vi "COPD_labview.vi"() -> ()   [LabVIEW 2022 SP3]
uses:
  <vilib>/DAQmx/read.llb/DAQmx Read (Analog DBL 1Chan 1Samp).vi
  <vilib>/Instr/_visa.llb/VISA Configure Serial Port (Instr).vi
  <vilib>/DAQmx/create/channels.llb/DAQmx Create Channel (AI-Voltage-Basic).vi
  <vilib>/DAQmx/miscellaneous.llb/DAQmx Fill In Error Info.vi
panel:
  out "Visa out":string
  out "Centered Piezo Chart":dbl(graph)
  in  "Peizo Baseline":dbl
  out "Command Sent":string
  in  "ESP32 COM Port":refnum<visa-resource-name>
  out "Bed Motor ON":bool
  out "Oxygen Relay ON":bool
  out "SpO2 Danger":bool
  out "Oxygen Required":bool
  in  "Danger Threshold":dbl
  out "SpO2 Chart":dbl(graph)
  out "SpO2  (%)":dbl
  in  "Oxygen Threshold":dbl
  out "Fever Alert":bool
  in  "Temperature Threshold":dbl
  out "Temperature(C) Indicator":dbl
  out "Temperature Chart":dbl(graph)
  in  "Breath Threshold":dbl
  in  "stop":bool
  out "Breath Detected":bool
  out "Piezo Signal Chart":dbl(graph)
  out "Respiratory Rate":dbl
  out "Piezo Voltage":dbl
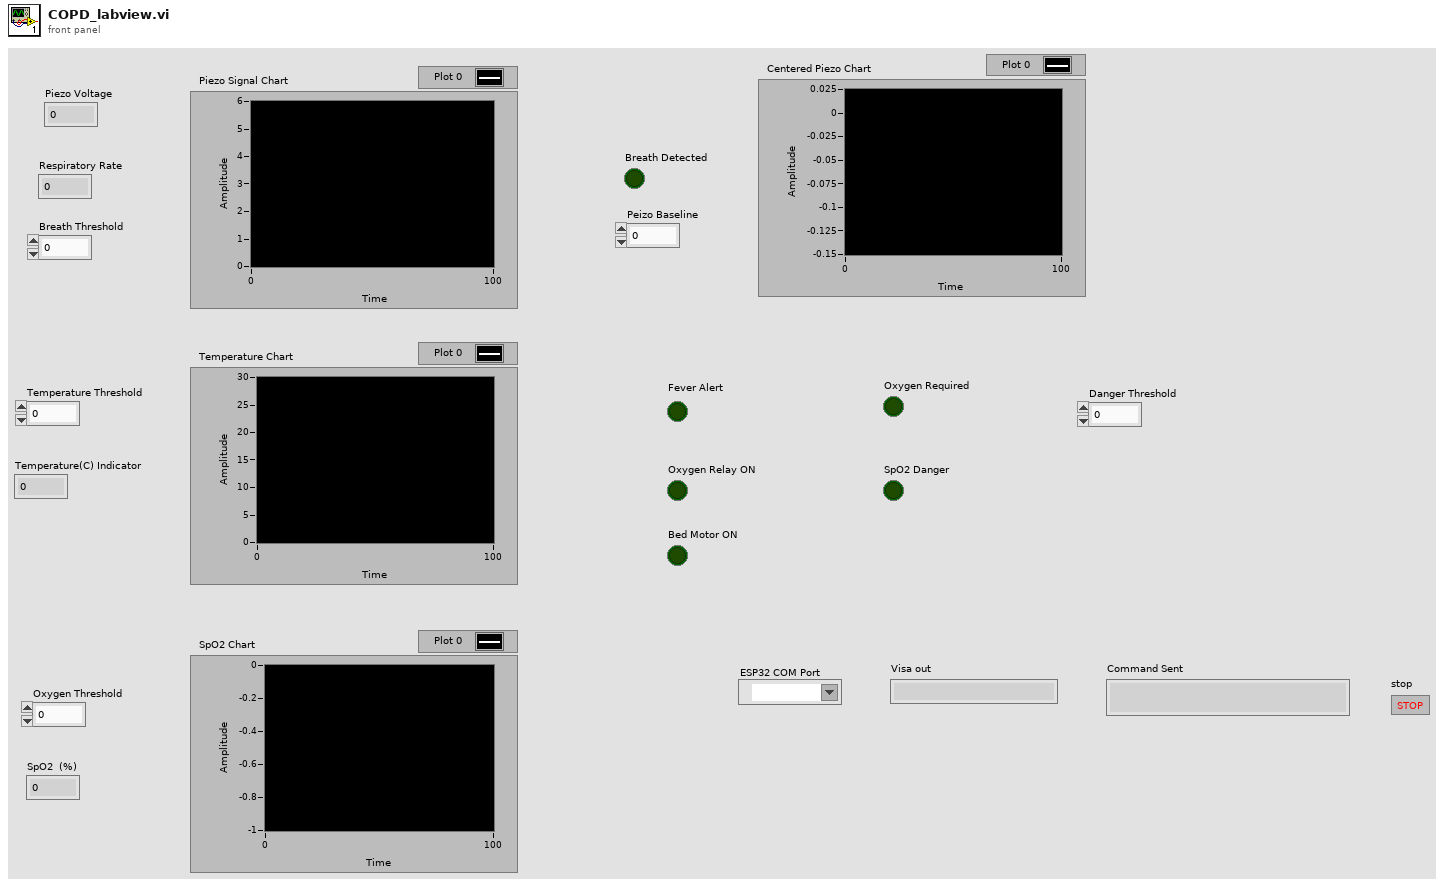
[diagram p1: front panel]
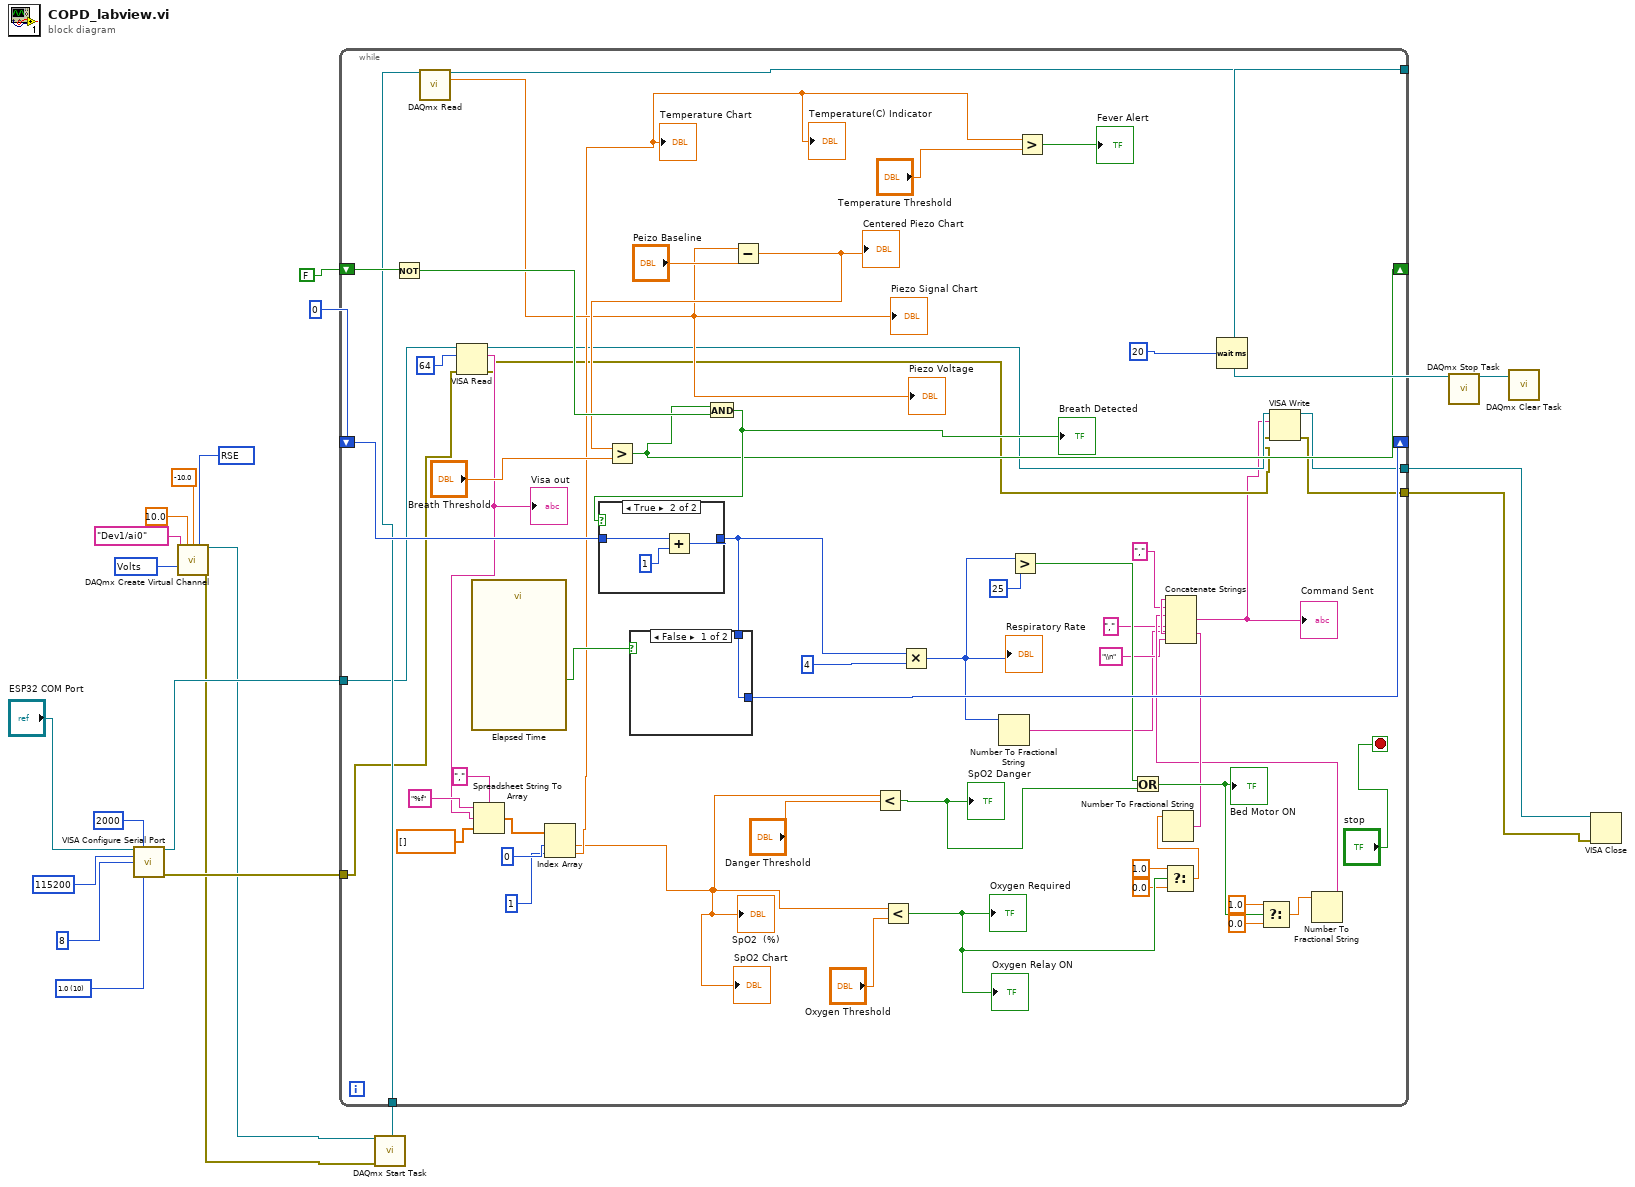
[diagram p0: block diagram]
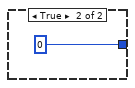
[diagram p2: hidden frame]
diagram:
  w7 = 10083 items=["Default"=-1, "RSE"=10083, "NRSE"=10078, "Differential"=10106, "Pseudodifferential"=12529] ("input terminal configuration")
  w10 = 10348 items=["Volts"=10348, "From Custom Scale"=10065] ("units")
  w14 = u16 10 items=["1.0"=10, "1.5"=15, "2.0"=20] ("stop bits (10: 1 bit)")
  n1 = call-poly "VISA Configure Serial Port"("VISA resource name"="ESP32 COM Port", "timeout (10sec)"=u32 2000, "baud rate (9600)"=u32 115200, "data bits (8)"=u16 8, "stop bits (10: 1 bit)"=w14) -> ("VISA resource name out"=w6:refnum<visa-resource-name>, "error out"=w12:errorcluster)  [unwired: 9 in]
  n2 = call-poly <vilib>:"DAQmx Create Virtual Channel.vi"("maximum value"=10.0, "minimum value"=-10.0, "input terminal configuration"=w7, "physical channels"=tag "Dev1/ai0", "units"=w10) -> ("task out"=w2:refnum<k21>, "error out"=w1:errorcluster)  [unwired: 9 in]
  n3 = call <vilib>:"DAQmx Start Task.vi"("task/channels in"=w2, "error in"=w1) -> ("task out"=w17:refnum<k21>)  [unwired: 12 in, 1 out]
  n4 = while {
    shift-right: [w49] -> _
    shift-left: FALSE -> [w76]
    shift-right: [w71] -> _
    shift-left: 0 -> [w74]
    tunnel: w17 -> [w67]
    tunnel: [w66] -> w19
    tunnel: w6 -> [w47]
    tunnel: w12 -> [w39]
    tunnel: [w32] -> w3
    tunnel: [w33] -> w4
    stop <- "stop" stop-if-true
    n5 = Not(x=w76) -> (.not. x?=w75:bool)
    n6 = call-poly <vilib>:"DAQmx Read.vi"("task/channels in"=w67) -> ("task out"=w66:refnum<k21>, "data"=w48:dbl)  [unwired: 12 in, 1 out]
    "Piezo Signal Chart" <- w48
    "Piezo Voltage" <- w48
    n7 = VISA Read(VISA resource name=w47, byte count=u32 64, error in (no error)=w39) -> (VISA resource name out=w35:refnum<visa-resource-name>, read buffer=w38:string, error out=w34:errorcluster)  [unwired: 1 out]
    "Visa out" <- w38
    n8 = call "Elapsed Time"() -> ("Time has Elapsed"=w72:bool)  [unwired: 12 in, 7 out]
    n9 = Spreadsheet String To Array(delimiter (Tab)=",", format string="%f", spreadsheet string=w38, array type (2D Dbl)=dbl[] []) -> (array=w37:dbl[])
    n10 = Index Array(array=w37, index #1=0 ("index"), index #2=1 ("index")) -> (element #1=w36:dbl, element #2=w42:dbl)
    "Temperature Chart" <- w42
    "Temperature(C) Indicator" <- w42
    "SpO2 Chart" <- w36
    "SpO2  (%)" <- w36
    n11 = Subtract(x=w48, y="Peizo Baseline") -> (x-y=w51:dbl)
    "Centered Piezo Chart" <- w51
    n12 = Greater?(x=w51, y="Breath Threshold") -> (0:w49:bool)
    n13 = And(x=w49, y=w75) -> (x .and. y?=w50:bool)
    "Breath Detected" <- w50
    n14 = case shown="True" w50 {
      tunnel: w74 -> [w80 w83]
      tunnel: [w80 w81] -> w70
      frame False {
      }
      frame True {
        n15 = Add(x=w83, y=1) -> (x+y=w81:i32)
      }
    }
    n16 = case shown="False" w72 {
      tunnel: [w78 0] -> w71
      tunnel: w70 -> [w78 _]
      frame False {
      }
      frame True {
      }
    }
    n17 = Less?(x=w36, y="Danger Threshold") -> (x < y?=w59:bool)
    "SpO2 Danger" <- w59
    n18 = Less?(x=w36, y="Oxygen Threshold") -> (x < y?=w58:bool)
    "Oxygen Required" <- w58
    "Oxygen Relay ON" <- w58
    n19 = Multiply(x=w70, y=4) -> (x*y=w23:i32)
    "Respiratory Rate" <- w23
    n20 = Number To Fractional String(number=w23) -> (F-format string=w22:string)  [unwired: 3 in]
    n21 = Greater?(x=w23, y=25) -> (0:w60:bool)
    n22 = Greater?(x=w42, y="Temperature Threshold") -> (0:→"Fever Alert":bool)
    n23 = Or(x=w60, y=w59) -> (x .or. y?=w55:bool)
    "Bed Motor ON" <- w55
    n24 = Select(t=1.0, s=w58, f=0.0) -> (s? t:f=w30:dbl)
    n25 = Number To Fractional String(number=w30) -> (F-format string=w29:string)  [unwired: 3 in]
    n26 = Wait (ms)(milliseconds to wait=20) -> ()  [unwired: 1 out]
    n27 = Select(t=1.0, s=w55, f=0.0) -> (s? t:f=w31:dbl)
    n28 = Number To Fractional String(number=w31) -> (F-format string=w27:string)  [unwired: 3 in]
    n29 = Concatenate Strings(w29, ",", w27, ",", w22, "\\n") -> (w26:string)
    "Command Sent" <- w26
    n30 = VISA Write(VISA resource name=w35, write buffer=w26, error in (no error)=w34) -> (VISA resource name out=w32:refnum<visa-resource-name>, error out=w33:errorcluster)  [unwired: 1 out]
  }
  n31 = call <vilib>:"DAQmx Stop Task.vi"("task/channels in"=w19) -> ("task out"=w18:refnum<k21>)  [unwired: 13 in, 1 out]
  n32 = call <vilib>:"DAQmx Clear Task.vi"("task in"=w18) -> ()  [unwired: 14 in, 1 out]
  n33 = VISA Close(VISA resource name=w3, error in (no error)=w4) -> ()  [unwired: 1 out]
